vi "Close Library Reference.vi"(8 "error in":errorcluster, 11 "Library Owner Reference":refnum<vi>) -> (0 "error out":errorcluster)   [LabVIEW 2022 SP3]
doc: "This VI closes the Library reference of the lvlib or lvclass that owns the User VI.\n\nIn this VI library means both lvlib and lvclass.\n\nError behaviour: Execute even if input error"
panel:
  # "Development\ncontrols/indicators useful for development and testing, but which are not outputs of the VI"
  # "Input\nInputs to the VI"
  # "Output\nOutputs of the VI"
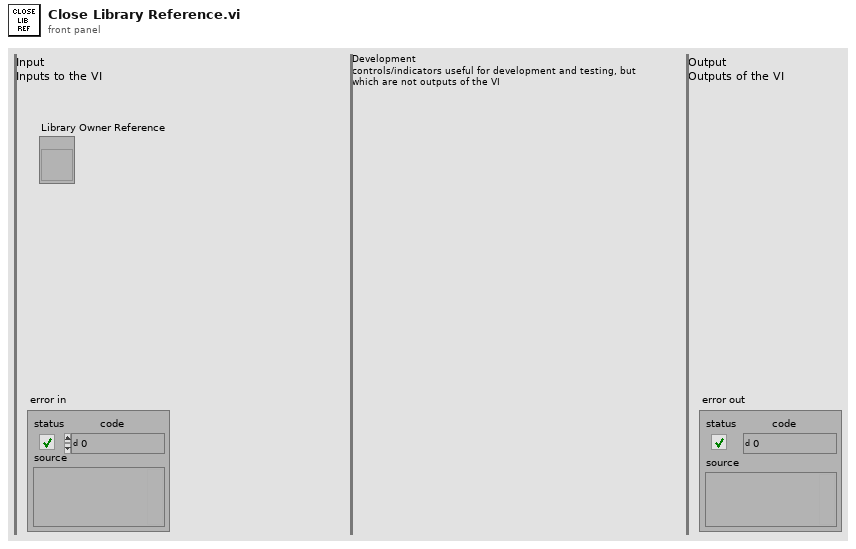
[diagram p1: front panel]
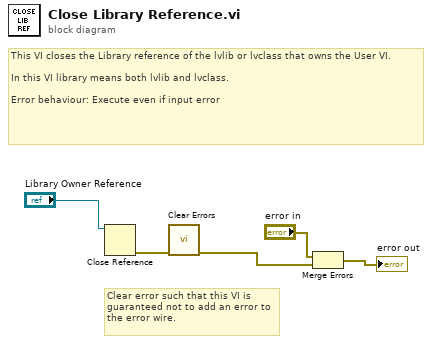
[diagram p0: block diagram]
diagram:
  # "Clear error such that this VI is guaranteed not to add an error to the error wire."
  # "This VI closes the Library reference of the lvlib or lvclass that owns the User VI.\n\nIn this VI library means both lvlib and lvclass.\n\nError behaviour: Execute even if input error"
  n1 = Close Reference(reference="Library Owner Reference") -> (error out=w5:errorcluster)  [unwired: 1 in]
  n2 = call <vilib>:"Clear Errors.vi"("error in (no error)"=w5) -> ("error out"=w1:errorcluster)  [unwired: 5 in, 1 out]
  n3 = Merge Errors("error in", w1) -> (→"error out":errorcluster)
